vi "Get RTPath String Array.vi"(8 "error in (no error)":errorcluster, 11 "Target OS":string) -> (0 "error out":errorcluster, 2 "File Path String Array":string[](array[string]), 3 "Target OS out":string)   [LabVIEW 2019, in "TLCD System Tests.lvclass"]
uses:
  TLCD System Tests.lvclass
  Source/System Explorer/Telemetry System Explorer.lvlib
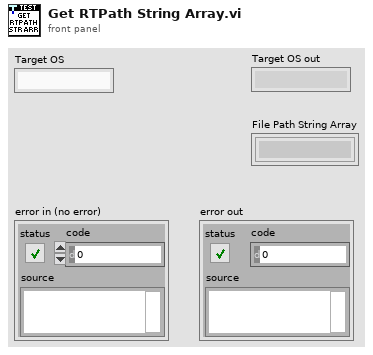
[diagram p1: front panel]
types:
  T1 = enum16{"PharLap", "VxWorks", "Windows", "Linux_32_ARM", "Linux_x64"}
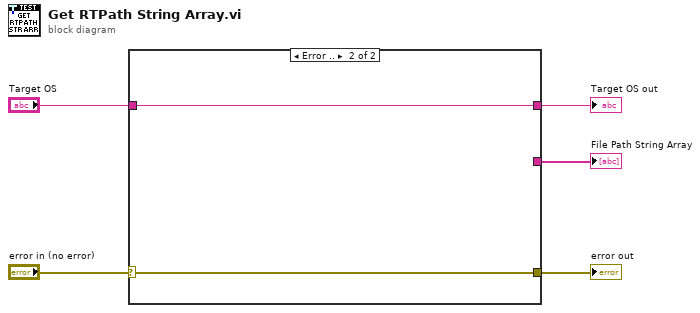
[diagram p0: block diagram]
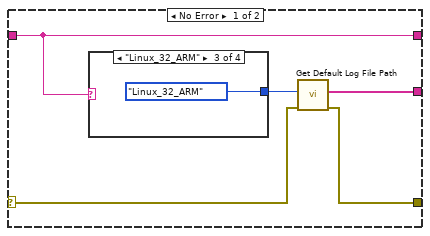
[diagram p2: hidden frame]
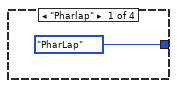
[diagram p3: hidden frame]
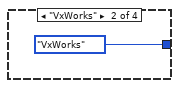
[diagram p4: hidden frame]
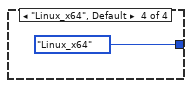
[diagram p5: hidden frame]
diagram:
  n1 = case shown="Error .." "error in (no error)" {
    selector: "error in (no error)" -> [w7 w15]
    tunnel: [w9 w15] -> w5
    tunnel: [w8 _] -> w4
    tunnel: "Target OS" -> [w6 w16]
    tunnel: [w6 w16] -> w1
    frame No Error {
      n2 = case shown="\"Linux_32_ARM\"" w6 {
        tunnel: [T1."PharLap" ("Target Type") T1."VxWorks" ("Target Type") T1."Linux_32_ARM" ("Target Type") T1."Linux_x64" ("Target Type")] -> w10
        frame "Pharlap" {
        }
        frame "VxWorks" {
        }
        frame "Linux_32_ARM" {
        }
        frame "Linux_x64", Default {
        }
      }
      n3 = call "Get Default Log File Path.vi"("error in"=w7, "Target Type"=w10) -> ("error out"=w9:errorcluster, "Log File Path String Array"=w8:string[])  [unwired: 8 in]
    }
    frame Error {
    }
  }
  "error out" <- w5
  "File Path String Array" <- w4
  "Target OS out" <- w1
